vi "Obtain Request Events.vi"(8 "error in":errorcluster, 10 "Create New? (F)":bool) -> (0 "error out":errorcluster, 2 "My Singleton Module Request Events":T1)   [LabVIEW 2020, in "My Singleton Module.lvlib"]
doc: "This VI Obtains/Creates the Requests events that will be used for other modules to communicate with the module that owns this VI. These Requests events will be accessed only via Public API methods for this module.\n\n<b>NOTE</b>: The contents of this VI are automatically generated and modified by the <b>Tools > DQMH Consortium > DQMH</b> utilities. Consider using those utilities instead of making your own modifications to this VI.\n_____\nBased on DQMH Project Template 7.1.0.1447."
uses:
  My Singleton Module.lvlib
  Request Events--cluster.ctl
  Stop Argument--cluster.ctl
  Do Something Argument--cluster.ctl
  Do Something Else Argument--cluster.ctl
  Do Something Else and Wait for Reply Argument--cluster.ctl
  Do Something Else and Wait (Reply Payload)--cluster.ctl
  Show Panel Argument--cluster.ctl
  Hide Panel Argument--cluster.ctl
  Get Module Execution Status Argument--cluster.ctl
  Show Diagram Argument--cluster.ctl
panel:
  # "NOTE: The contents of this VI are automatically generated and modified by the Tools > DQMH Consortium > DQMH utilities. Consider using those utilities instead of making your own modifications to this VI."
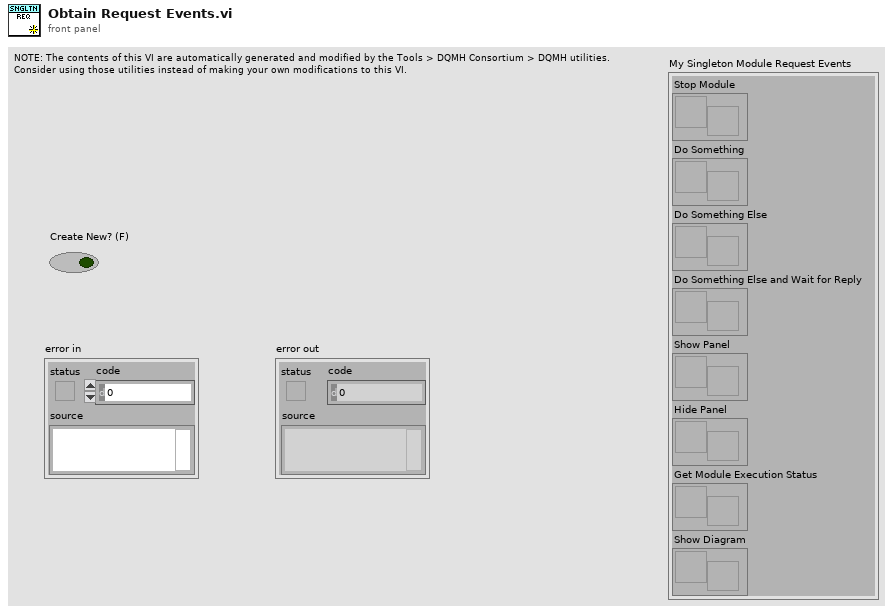
[diagram p1: front panel]
types:
  T1 = typedef "My Singleton Module.lvlib/Request Events--cluster.ctl" = cluster{"Stop Module":refnum<user-event>, "Do Something":refnum<user-event>, "Do Something Else":refnum<user-event>, "Do Something Else and Wait for Reply":refnum<user-event>, "Show Panel":refnum<user-event>, "Hide Panel":refnum<user-event>, "Get Module Execution Status":refnum<user-event>, "Show Diagram":refnum<user-event>}
  T2 = typedef "My Singleton Module.lvlib/Hide Panel Argument--cluster.ctl" = cluster{"Hide Panel?":bool}
  T3 = typedef "My Singleton Module.lvlib/Show Panel Argument--cluster.ctl" = cluster{"Show Panel?":bool}
  T4 = typedef "My Singleton Module.lvlib/Show Diagram Argument--cluster.ctl" = cluster{"Debug?":bool}
  T5 = typedef "My Singleton Module.lvlib/Get Module Execution Status Argument--cluster.ctl" = cluster{"Running?":bool}
  T6 = typedef "My Singleton Module.lvlib/Do Something Else and Wait for Reply Argument--cluster.ctl" = cluster{"Do Something Else Msg":string, "X":dbl, "Wait Notifier":refnum<notifier>, "wait for reply":bool}
  T7 = typedef "My Singleton Module.lvlib/Do Something Else Argument--cluster.ctl" = cluster{"Do Something Else Msg":string, "X":dbl}
  T8 = typedef "My Singleton Module.lvlib/Do Something Argument--cluster.ctl" = cluster{"Do Something Msg":string}
  T9 = typedef "My Singleton Module.lvlib/Stop Argument--cluster.ctl" = cluster{"Origin":string, "Exit via Stop Module Req?":bool, "Wait for Module to stop?":bool}
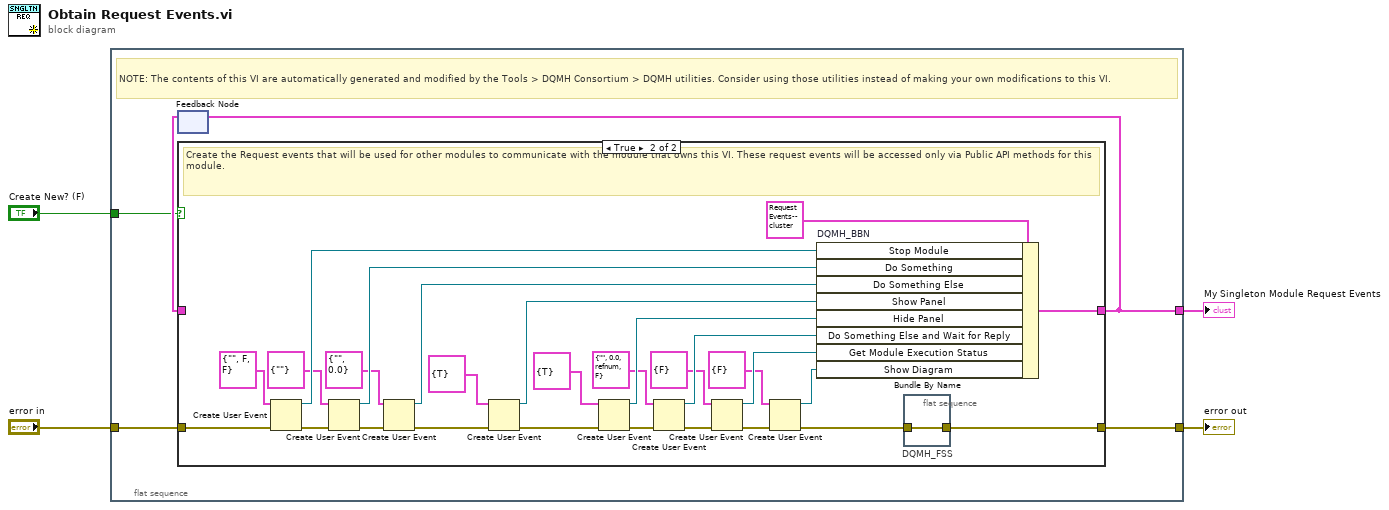
[diagram p0: block diagram]
diagram:
  n1 = flat-sequence {
    tunnel: [w9] -> w4
    tunnel: "error in" -> [w8]
    tunnel: [w6] -> w2
    tunnel: "Create New? (F)" -> [w5]
    frame #0 {
      # "NOTE: The contents of this VI are automatically generated and modified by the Tools > DQMH Consortium > DQMH utilities. Consider using those utilities instead of making your own modifications to this VI."
      n2 = feedback #1() -> (w7:T1)  [unwired: 1 in]
      n3 = case shown="True" w5 {
        tunnel: [w10 w20] -> w9
        tunnel: w8 -> [w10 w39]
        tunnel: [w11 w36] -> w6
        tunnel: w7 -> [w11 _]
        frame False {
          # "Obtain the Request events that were created in a previous call to this VI."
        }
        frame True {
          # "Create the Request events that will be used for other modules to communicate with the module that owns this VI. These request events will be accessed only via Public API methods for this module."
          n4 = Create User Event(user event datatype=T9 {"Origin"="", "Exit via Stop Module Req?"=FALSE, "Wait for Module to stop?"=FALSE} ("Stop Argument"), error in=w39) -> (user event=w37:refnum<user-event>, error out=w33:errorcluster)
          n5 = Create User Event(user event datatype=T8 {"Do Something Msg"=""} ("Do Something Argument"), error in=w33) -> (user event=w32:refnum<user-event>, error out=w31:errorcluster)
          n6 = Create User Event(user event datatype=T7 {"Do Something Else Msg"="", "X"=0.0} ("Do Something Else Argument"), error in=w31) -> (user event=w29:refnum<user-event>, error out=w28:errorcluster)
          n7 = Create User Event(user event datatype=T3 {"Show Panel?"=TRUE} ("Show Panel Argument"), error in=w28) -> (user event=w27:refnum<user-event>, error out=w26:errorcluster)
          n8 = Create User Event(user event datatype=T2 {"Hide Panel?"=TRUE} ("Hide Panel Argument"), error in=w26) -> (user event=w25:refnum<user-event>, error out=w24:errorcluster)
          n9 = Create User Event(user event datatype=T6 {"Do Something Else Msg"="", "X"=0.0, "Wait Notifier"=refnum, "wait for reply"=FALSE} ("Do Something Else and Wait for Reply Argument"), error in=w24) -> (user event=w23:refnum<user-event>, error out=w21:errorcluster)
          n10 = Create User Event(user event datatype=T5 {"Running?"=FALSE} ("Get Module Execution Status Argument"), error in=w21) -> (user event=w18:refnum<user-event>, error out=w19:errorcluster)
          n11 = Create User Event(user event datatype=T4 {"Debug?"=FALSE} ("Show Diagram Argument"), error in=w19) -> (user event=w15:refnum<user-event>, error out=w16:errorcluster)
          n12 = Bundle By Name "DQMH_BBN"(cluster=T1 {"Stop Module"=refnum, "Do Something"=refnum, "Do Something Else"=refnum, "Do Something Else and Wait for Reply"=refnum, "Show Panel"=refnum, "Hide Panel"=refnum, "Get Module Execution Status"=refnum, "Show Diagram"=refnum} ("output cluster"), "Stop Module"=w37, "Do Something"=w32, "Do Something Else"=w29, "Show Panel"=w27, "Hide Panel"=w25, "Do Something Else and Wait for Reply"=w23, "Get Module Execution Status"=w18, "Show Diagram"=w15) -> (w36:T1)
          n13 = flat-sequence "DQMH_FSS" {
            tunnel: w16 -> [w40]
            tunnel: [w40] -> w20
            frame #0 {
            }
          }
        }
      }
      n14 = feedback-in #1(w6) -> ()
    }
  }
  "My Singleton Module Request Events" <- w2
  "error out" <- w4
